vi "总磷总氮流程质控自动启动.vi"(9 "总磷量程切换":enum32{"H", "L", "AUTO"}(ring)=enum."AUTO", 10 "总氮量程切换":enum32{"H", "L", "AUTO"}(ring)=enum."AUTO", 11 "参数":T1={"是否启用仪器"=FALSE, "CODMn"={"启动测量模式"={"测量模式"=enum."水样测量"}, "确定按钮"=TRUE}, "启动模块"={"氨氮"=FALSE, "总磷"=FALSE, "总氮"=FALSE, "COD"=FALSE}, "常规启动"=FALSE, "直接启动"=FALSE}) -> ()   [LabVIEW 2016, in "质控单元.lvlib"]
panel:
  out "枚举 2":enum16{"初始化", "采配水启动", "等待", "配水", "排水", "结束"}(ring)
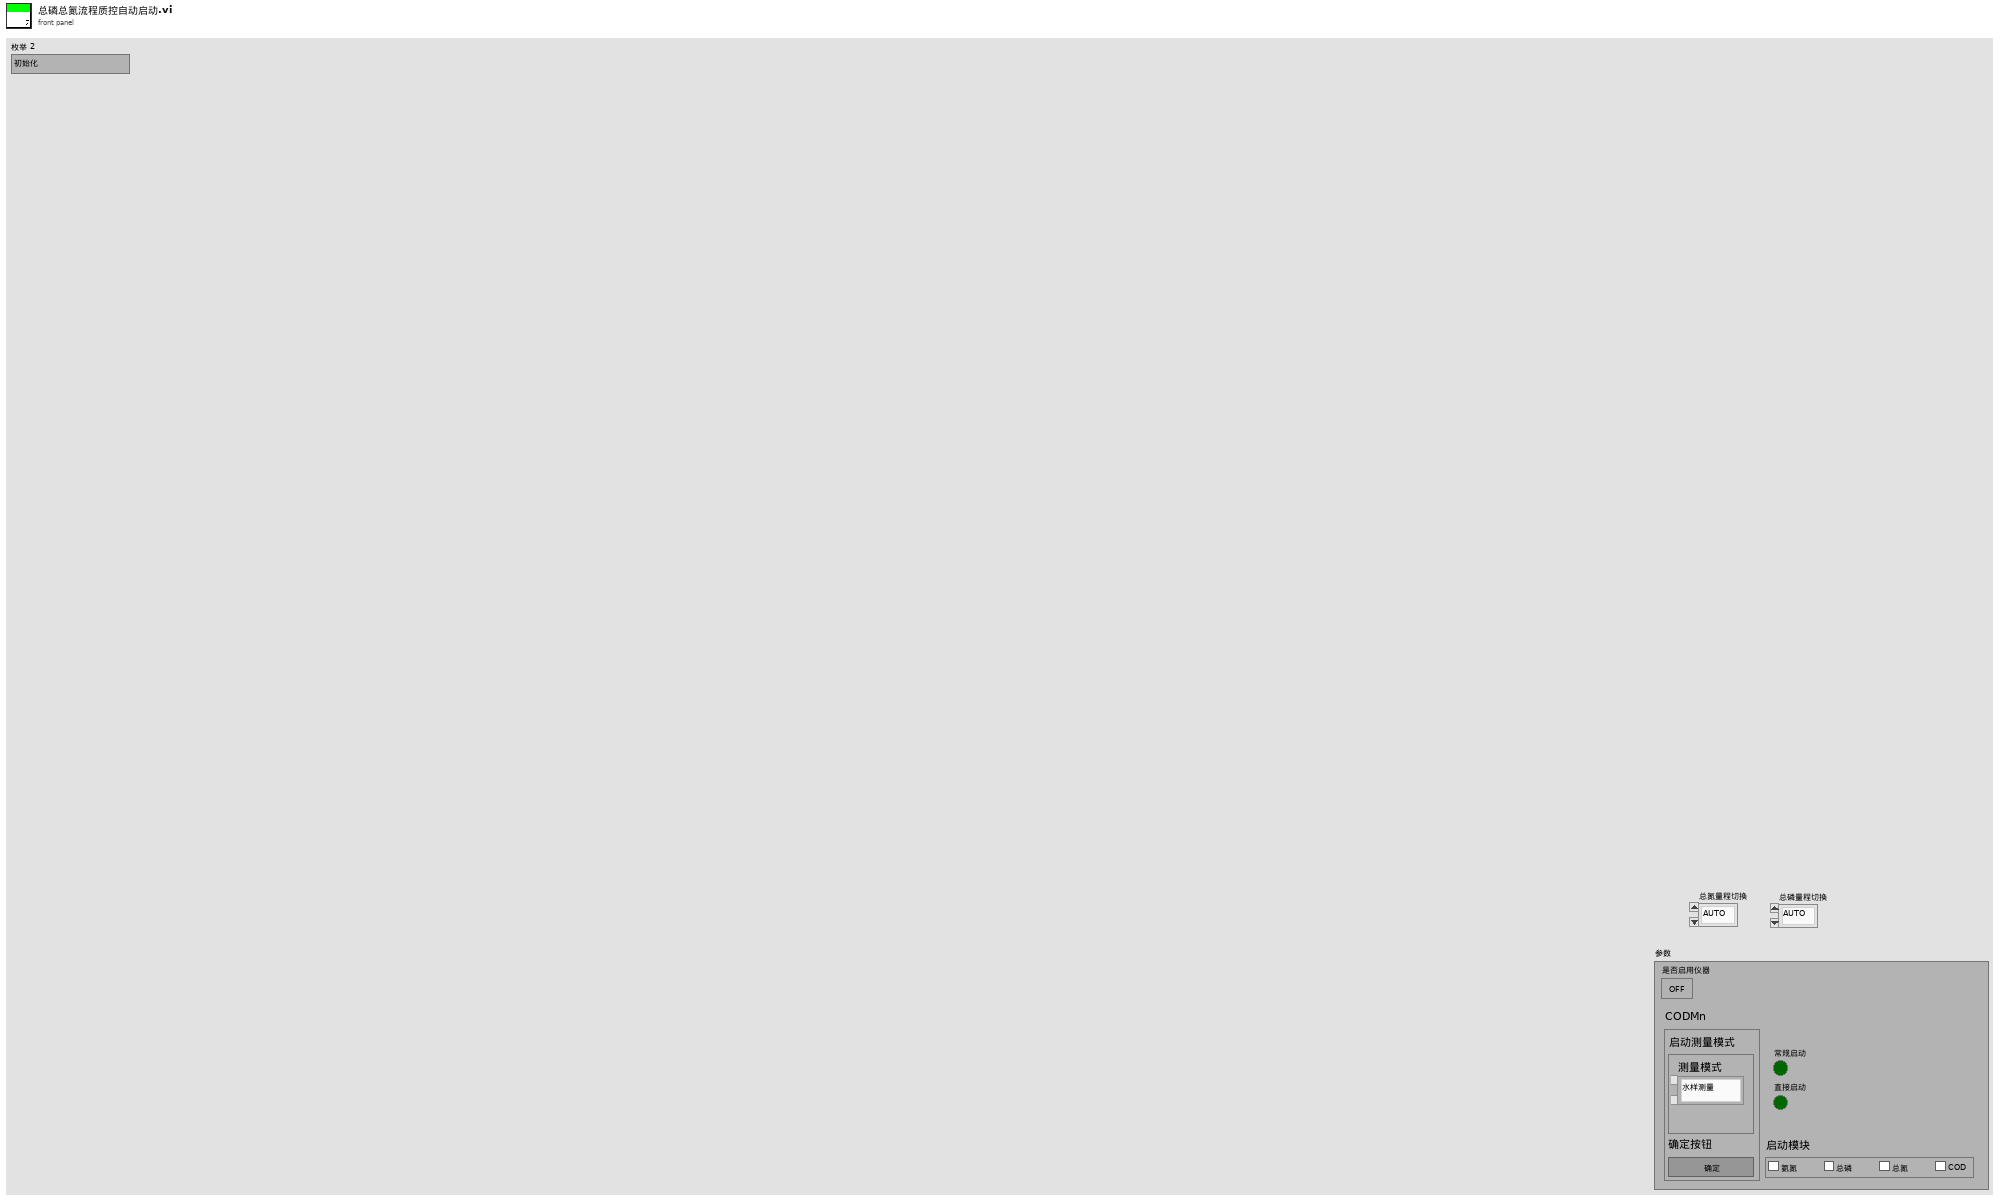
[diagram p1: front panel]
types:
  T1 = cluster{"是否启用仪器":bool, "CODMn":cluster{"启动测量模式":cluster{"测量模式":enum16{"水样测量", "标样核查", "加标回收", "平行样", "校零", "校标"}}, "确定按钮":bool}, "启动模块":cluster{"氨氮":bool, "总磷":bool, "总氮":bool, "COD":bool}, "常规启动":bool, "直接启动":bool}
  T2 = cluster{"R0":i16, "R1":i16, "R2":i16, "R3":i16, "R4":i16, "R5":i16, "R6":i16, "R7":i16, "R8":i16, "R9":i16, "R10":i16, "R11":i16, "R12":i16, "R13":i16, "R14":i16, "R15":i16, "R16":i16, "R17":i16, "R18":i16, "R19":i16, "R20":i16, "R21":i16, "R22":i16, "R23":i16, "R24":i16, "R25":i16, "R26":i16, "R27":i16, "R28":i16, "R29":i16, "R30":i16, "R31":i16, "R32":i16, "R33":i16, "R34":i16, "R35":i16, "R36":i16, "R37":i16, "R38":i16, "R39":i16, "R40":i16, "R41":i16, "R42":i16, "R43":i16, "R44":i16, "R45":i16, "R46":i16, "R47":i16, "R48":i16, "R49":i16, "R50":i16, "R51":i16, "R52":i16, "R53":i16, "R54":i16, "R55":i16, "R56":i16}
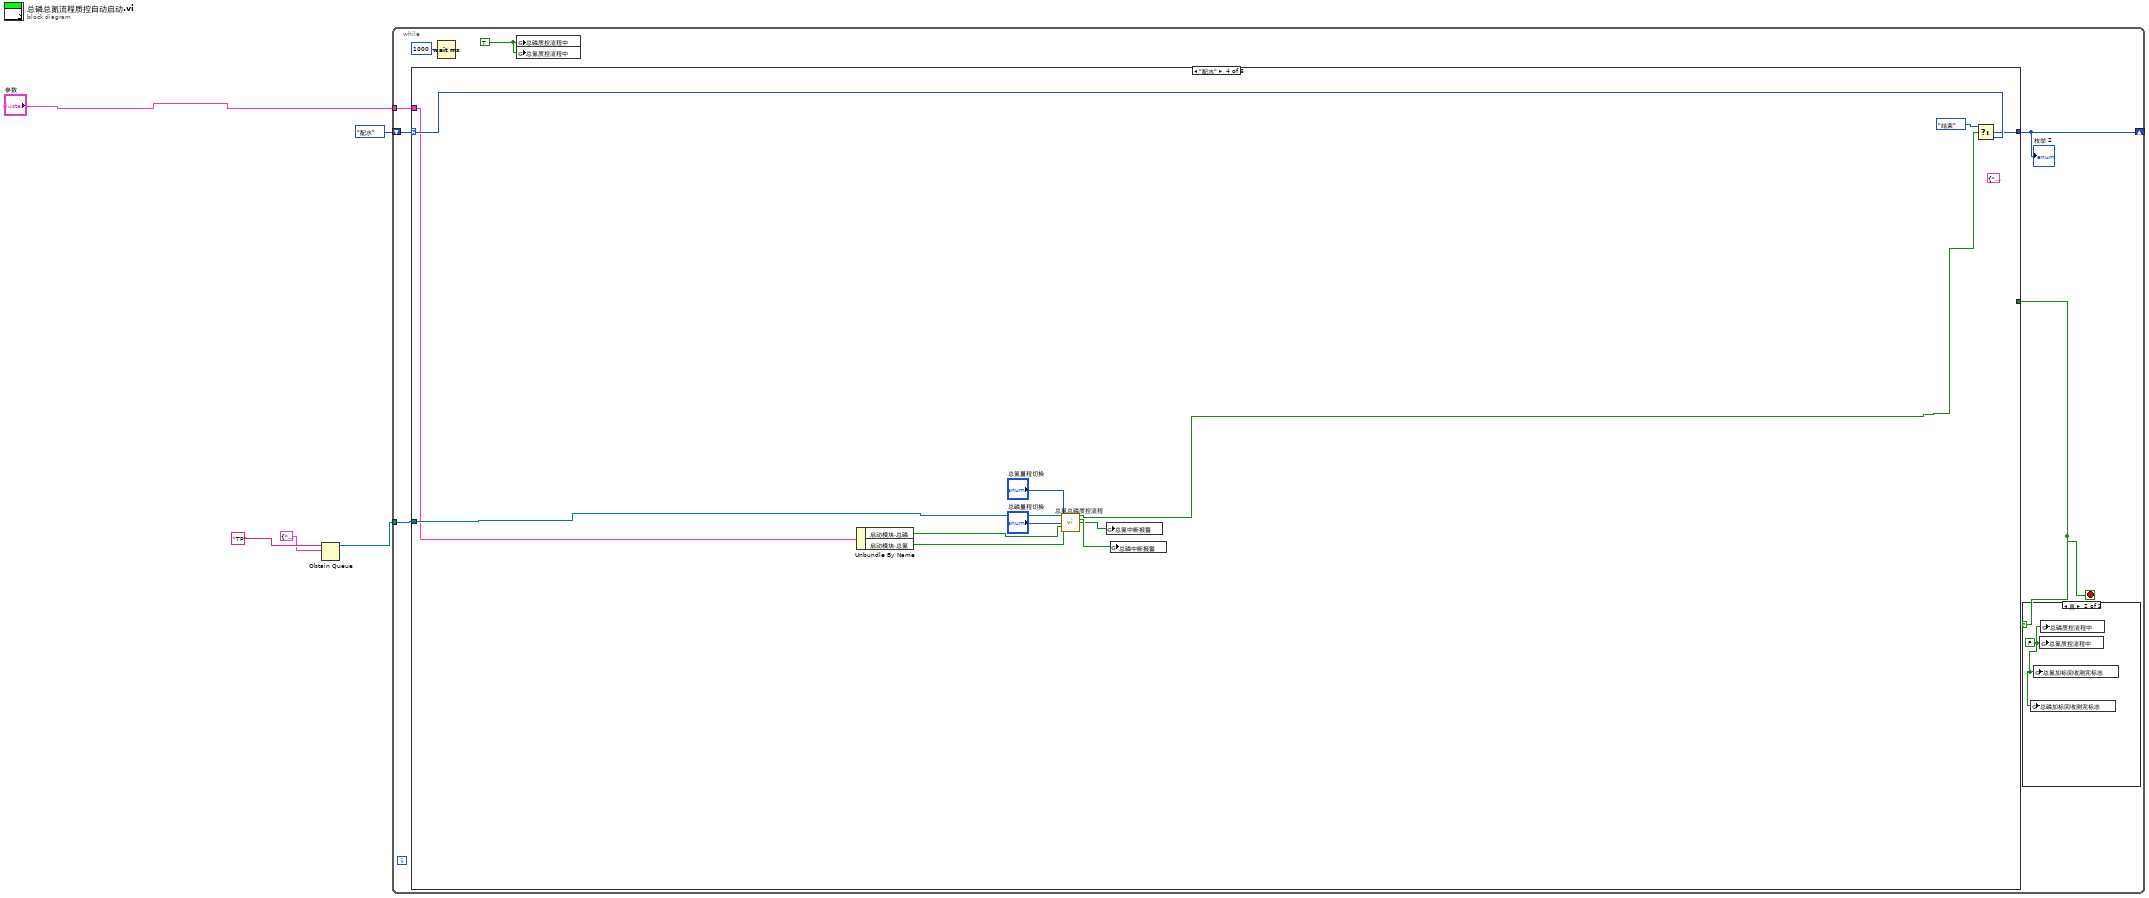
[diagram p0: block diagram]
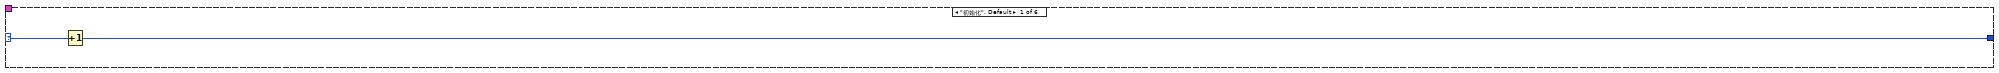
[diagram p3: hidden frame]
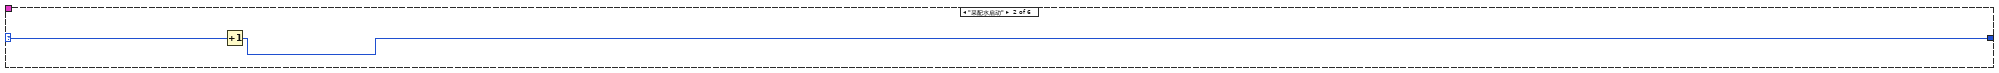
[diagram p4: hidden frame]
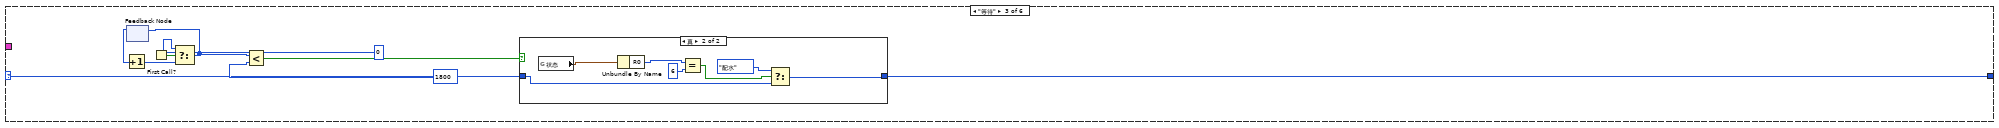
[diagram p5: hidden frame]
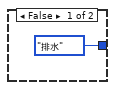
[diagram p6: hidden frame]
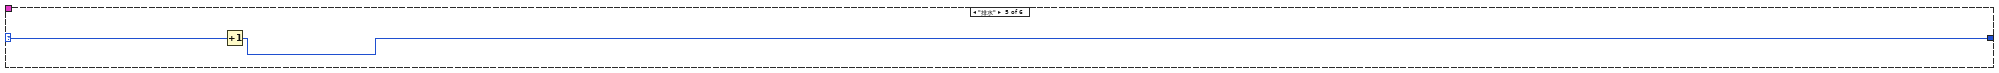
[diagram p7: hidden frame]
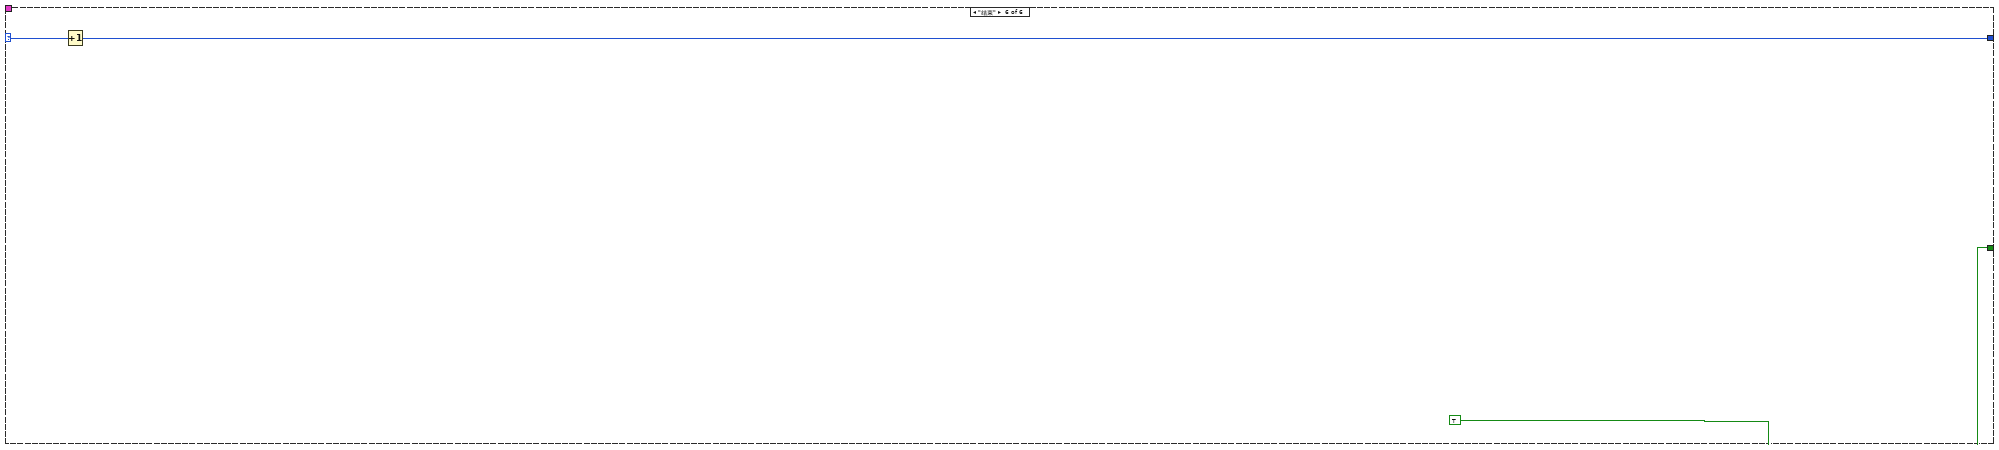
[diagram p8: hidden frame]
diagram:
  n1 = Obtain Queue(name (unnamed)="TP" ("名称（未命名）"), element data type=cluster{"命令":string, "data":variant} {"命令"="", "data"=variant}) -> (queue out=w1:refnum<queue>)  [unwired: 3 in, 2 out]
  n2 = while {
    shift-right: [w11] -> _
    shift-left: enum16{"初始化", "采配水启动", "等待", "配水", "排水", "结束"}."配水" ("枚举") -> [w12]
    tunnel: w1 -> [w9]
    tunnel: "参数" -> [w8]
    stop <- w6 stop-if-true
    w7 = TRUE ("总磷质控流程中")
    n3 = case shown="\"配水\"" w12 {
      selector: w12 -> [w15 w17 w24 w45 w48 w51]
      tunnel: [w14 w16 w23 w44 w47 w50] -> w11
      tunnel: [_ _ _ _ _ TRUE] -> w6
      tunnel: w9 -> [_ _ _ w43 _ _]
      tunnel: w8 -> [_ _ _ w37 _ _]
      frame "初始化", Default {
        n4 = Increment(x=w15) -> (x+1=w14:enum16{"初始化", "采配水启动", "等待", "配水", "排水", "结束"})
      }
      frame "采配水启动" {
        n5 = Increment(x=w17) -> (x+1=w16:enum16{"初始化", "采配水启动", "等待", "配水", "排水", "结束"})
      }
      frame "等待" {
        n6 = feedback #1() -> (w20:i32)  [unwired: 1 in]
        n7 = Increment(x=w20) -> (x+1=w19:i32)
        n8 = First Call?() -> (First Call?: T/F=w21:bool)
        n9 = Select(t=0, s=w21, f=w19) -> (s? t:f=w18:i32)
        n10 = feedback-in #1(w18) -> ()
        n11 = Less?(x=w18, y=1800) -> (x < y?=w25:bool)
        n12 = case shown="真" w25 {
          tunnel: w24 -> [_ w30]
          tunnel: [enum16{"初始化", "采配水启动", "等待", "配水", "排水", "结束"}."排水" ("枚举") w29] -> w23
          frame False {
          }
          frame True {
            n13 = global read "与采配水交互全局.vi" "状态"() -> (w28:T2)
            n14 = Unbundle By Name(w28) -> ("R0"=w34:i16)
            n15 = Equal?(x=w34, y=i16 6) -> (x = y?=w32:bool)
            n16 = Select(t=enum16{"初始化", "采配水启动", "等待", "配水", "排水", "结束"}."配水" ("枚举"), s=w32, f=w30) -> (s? t:f=w29:enum16{"初始化", "采配水启动", "等待", "配水", "排水", "结束"})
          }
        }
      }
      frame "配水" {
        (unwired) cluster{"命令":string, "data":variant} {"命令"="启动", "data"=variant(cluster{"站号":u16, "控制命令输出":u16[]} {"站号"=1, "控制命令输出"=[256, 0]})} ("元素")
        n17 = Unbundle By Name(w37) -> ("启动模块.总磷"=w36:bool, "启动模块.总氮"=w35:bool)
        n18 = call "总氮总磷质控流程.vi"("队列输入TP"=w43, "总氮量程切换"="总氮量程切换", "总磷量程切换"="总磷量程切换", "总磷"=w36, "总氮"=w35) -> ("布尔"=w40:bool, "总磷中断报警"=w39:bool, "总氮中断报警"=w38:bool)  [unwired: 8 in]
        n19 = global write "质控中断报警全局.vi" "总氮中断报警"(w38) -> ()
        n20 = global write "质控中断报警全局.vi" "总磷中断报警"(w39) -> ()
        n21 = Select(t=enum16{"初始化", "采配水启动", "等待", "配水", "排水", "结束"}."结束" ("枚举"), s=w40, f=w45) -> (s? t:f=w44:enum16{"初始化", "采配水启动", "等待", "配水", "排水", "结束"})
      }
      frame "排水" {
        n22 = Increment(x=w48) -> (x+1=w47:enum16{"初始化", "采配水启动", "等待", "配水", "排水", "结束"})
      }
      frame "结束" {
        n23 = Increment(x=w51) -> (x+1=w50:enum16{"初始化", "采配水启动", "等待", "配水", "排水", "结束"})
      }
    }
    "枚举 2" <- w11
    n24 = Wait (ms)(milliseconds to wait=u32 1000 ("等待时间（毫秒）")) -> ()  [unwired: 1 out]
    n25 = global write "质控测完标志全局 1.vi" "总磷质控流程中"(w7) -> ()
    n26 = global write "质控测完标志全局 1.vi" "总氮质控流程中"(w7) -> ()
    n27 = case shown="真" w6 {
      frame False {
      }
      frame True {
        w13 = FALSE ("总氮质控流程中")
        n28 = global write "质控测完标志全局 1.vi" "总磷加标回收测完标志"(w13) -> ()
        n29 = global write "质控测完标志全局 1.vi" "总氮加标回收测完标志"(w13) -> ()
        n30 = global write "质控测完标志全局 1.vi" "总氮质控流程中"(w13) -> ()
        n31 = global write "质控测完标志全局 1.vi" "总磷质控流程中"(w13) -> ()
      }
    }
  }
